vi "SV Cross Spectrum (Mag-Phase).vi"(0 "scaled signal X [EUx]":dbl[](array[numeric]) format="%.2f", 1 "window":T6=1 items=["None"=0, "Hanning"=1, "Hamming"=2, "Blackman-Harris"=3, "Exact Blackman"=4, "Blackman"=5, "Flat Top"=6, "4 Term B-Harris "=7, "7 Term B-Harris"=8, "Low Sidelobe"=9, "Force - Exponential"=10, "Blackman Nuttall"=11, "Triangle"=30, "Bartlett-Hanning"=31, "Bohman"=32, "Parzen"=33, "Welch"=34, "Kaiser"=60, "Dolph-Chebyshev"=61, "Gaussian"=62], 2 "force/exp settings":T5={"force window [%]"=50.0, "exponential window [%]"=10.0} {"exponential window [%]" min=0.0 max=100.0 format="%.2f"; "force window [%]" min=0.0 max=100.0 format="%.2f"}, 5 "scaled signal Y [EUy]":dbl[](array[numeric]) format="%.2f", 7 "sampling frequency [Hz]":dbl=10000.0 format="%.2f", 9 "channel X info":T1={"sensor sensitivity [mV/EU]"=1000.0, "engineering units"=1, "dB reference [EU]"=1.0, "custom label"="EU", "weighting filter"=0, "pregain [dB]"=0.0} {"pregain [dB]" format="%.2f"; "weighting filter" items=["Linear", "A-weighting", "B-weighting", "C-weighting", "ITU-R 468-4", "Dolby", "CCITT", "C-message"]; "dB reference [EU]" format="%^.1e"; "engineering units" items=["custom..."=0, "V"=1, "A"=21, "Pa"=2, "N"=20, "g"=3, "m/s^2"=4, "m/s"=5, "m"=6, "mm/s"=12, "mm"=13, "microns/s"=14, "microns"=15, "in/s^2"=7, "in/s"=8, "in"=9, "mils/s"=10, "mils"=11, "rad/s^2"=16, "rad/s"=17, "rad"=18, "strain"=19]; "sensor sensitivity [mV/EU]" format="%.2f"}, 11 "channel Y info":T1={"sensor sensitivity [mV/EU]"=1000.0, "engineering units"=1, "dB reference [EU]"=1.0, "custom label"="EU", "weighting filter"=0, "pregain [dB]"=0.0} {"pregain [dB]" format="%.2f"; "weighting filter" items=["Linear", "A-weighting", "B-weighting", "C-weighting", "ITU-R 468-4", "Dolby", "CCITT", "C-message"]; "dB reference [EU]" format="%^.1e"; "engineering units" items=["custom..."=0, "V"=1, "A"=21, "Pa"=2, "N"=20, "g"=3, "m/s^2"=4, "m/s"=5, "m"=6, "mm/s"=12, "mm"=13, "microns/s"=14, "microns"=15, "in/s^2"=7, "in/s"=8, "in"=9, "mils/s"=10, "mils"=11, "rad/s^2"=16, "rad/s"=17, "rad"=18, "strain"=19]; "sensor sensitivity [mV/EU]" format="%.2f"}, 12 "view":T4) -> (4 "magnitude [EUx EUy rms]":dbl[](array[numeric]) format="%.2f", 6 "unit label (magnitude)":string, 8 "phase":dbl[](array[numeric]) format="%.2f", 10 "unit label (phase)":string, 14 "window constants":cluster{"eq noise BW":dbl, "coherent gain":dbl} {"coherent gain" format="%.2f"; "eq noise BW" format="%.2f"}, 15 "df [Hz]":dbl format="%.2f")   [LabVIEW 2017]
doc: "SV (Sound & Vibration) Cross Spectrum (Mag-Phase) computes the cross power spectrum of the input signals. Typically, X signal is the stimulus, and Y signal is the response of the system. Results are returned as magnitude and phase.\nThe view cluster allows you to display magnitude results in decibels, and the phase results unwrapped or not, in radians or degrees."
uses:
  <vilib>/addons/_NISVFA/_Shared subVIs/Controls/svc_Window [Dual FFT].ctl
  <vilib>/addons/Sound and Vibration/compatibility/Controls/svl_Channel Info.ctl
  <vilib>/addons/Sound and Vibration/compatibility/Controls/svl_Engineering Units Text Ring.ctl
  <vilib>/addons/Sound and Vibration/compatibility/Controls/svl_Weighting Filter Text Ring.ctl
  <vilib>/Analysis/4window.llb/Force Window (DBL).vi
  <vilib>/Analysis/4window.llb/Exponential Window (DBL).vi
  <vilib>/Analysis/2dsp.llb/Cross Power (DBL).vi
  <vilib>/Analysis/0measdsp.llb/Scaled Time Domain Window (DBL).vi
  <vilib>/Analysis/NI_AALPro.lvlib
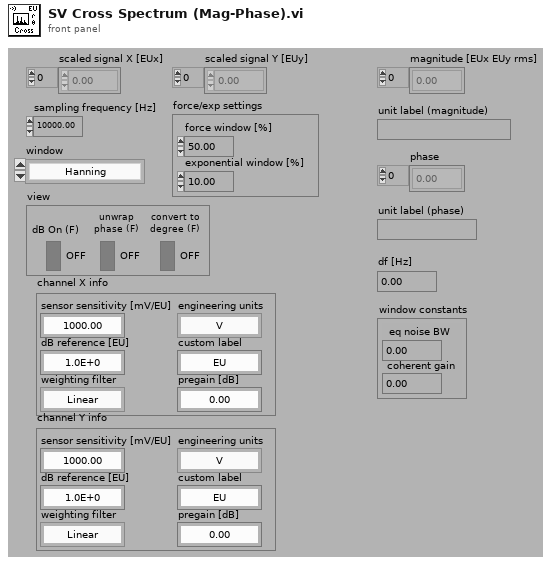
[diagram p1: front panel]
types:
  T1 = typedef "svl_Channel Info.ctl" = cluster{"sensor sensitivity [mV/EU]":dbl, "engineering units":T2, "dB reference [EU]":dbl, "custom label":string, "weighting filter":T3, "pregain [dB]":dbl}
  T2 = typedef "svl_Engineering Units Text Ring.ctl" = u16
  T3 = typedef "svl_Weighting Filter Text Ring.ctl" = u16
  T4 = cluster{"dB On (F)":bool, "unwrap phase (F)":bool, "convert to degree (F)":bool}
  T5 = cluster{"force window [%]":dbl, "exponential window [%]":dbl}
  T6 = typedef "svc_Window [Dual FFT].ctl" = u32
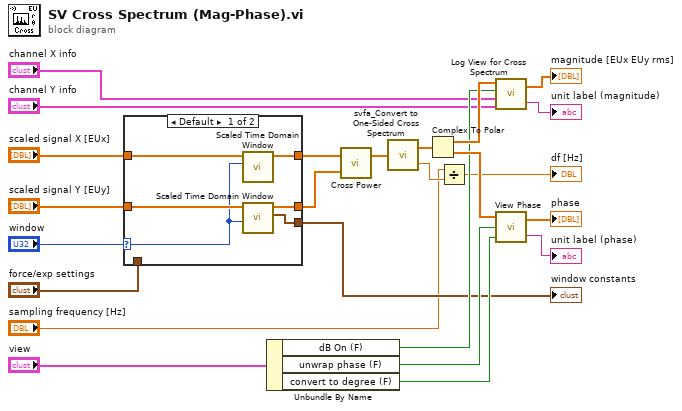
[diagram p0: block diagram]
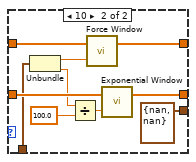
[diagram p2: hidden frame]
diagram:
  n1 = case shown="Default" "window" {
    selector: "window" -> [w25 _]
    tunnel: "scaled signal X [EUx]" -> [w30 w40]
    tunnel: "scaled signal Y [EUy]" -> [w29 w39]
    tunnel: "force/exp settings" -> [_ w35]
    tunnel: [w28 w37] -> w5
    tunnel: [w27 w36] -> w4
    tunnel: [w26 cluster{"eq noise BW":dbl, "coherent gain":dbl} {"eq noise BW"=nan, "coherent gain"=nan} ("window constants")] -> w10
    frame Default {
      n2 = call-poly <vilib>:"Scaled Time Domain Window.vi"("window"=w25, "X"=w30) -> ("Windowed X"=w28:dbl[])  [unwired: 7 in, 2 out]
      n3 = call-poly <vilib>:"Scaled Time Domain Window.vi"("window"=w25, "X"=w29) -> ("window properties"=w26:cluster{"eq noise BW":dbl, "coherent gain":dbl}, "Windowed X"=w27:dbl[])  [unwired: 7 in, 1 out]
    }
    frame 10 {
      n4 = Unbundle(w35) -> ("force window [%]"=w34:dbl, "exponential window [%]"=w33:dbl)
      n5 = Divide(x=w33, y=100.0 ("x")) -> (x/y=w38:dbl)
      n6 = call-poly <vilib>:"Force Window.vi"("duty cycle(%)"=w34, "X"=w40) -> ("Windowed X"=w37:dbl[])  [unwired: 1 out]
      n7 = call-poly <vilib>:"Exponential Window.vi"("final value"=w38, "X"=w39) -> ("Windowed X"=w36:dbl[])  [unwired: 1 out]
    }
  }
  "window constants" <- w10
  n8 = Unbundle By Name("view") -> ("dB On (F)"=w13:bool, "unwrap phase (F)"=w15:bool, "convert to degree (F)"=w14:bool)
  n9 = call-poly <vilib>:"Cross Power.vi"("Y"=w4, "X"=w5) -> ("Sxy"=w6:cdb[])  [unwired: 1 out]
  n10 = call <vilib>:"svfa_Convert to One-Sided Cross Spectrum.vi"("two-sided cross spectrum"=w6) -> ("one-sided cross spectrum"=w3:cdb[], "block size"=w7:dbl)
  n11 = Complex To Polar(r * e^(i*theta)=w3) -> (r=w17:dbl[], theta=w20:dbl[])
  n12 = Divide(x="sampling frequency [Hz]", y=w7) -> (x/y=→"df [Hz]":dbl)
  n13 = call <vilib>:"Log View for Cross Spectrum.vi"("channel Y info"="channel Y info", "channel X info"="channel X info", "dB On (T)"=w13, "cross spectrum [EUx EUy rms]"=w17) -> ("unit label"=→"unit label (magnitude)":string, "log view cross spectrum [dB EUx EUy]"=→"magnitude [EUx EUy rms]":dbl[])
  n14 = call <vilib>:"View Phase.vi"("convert to degree (F)"=w14, "unwrap phase (F)"=w15, "phase (radian)"=w20) -> ("unit label (phase)"=→"unit label (phase)":string, "scaled phase"=→"phase":dbl[])
